vi "ListBox_MultiListBox.vi"() -> ()   [LabVIEW 2025]
doc: "Converts a 2D array into a multi-column listbox by using both the 'ItemNames' and 'Headers' property nodes, and also converts a 1D array into a listbox using the 'ItemNames' property node, allowing the user to select a value from the list, and displays the selected value."
panel:
  out "String":string
  out "Numeric":i32
  in  "Array 4":string[](array[string])
  in  "Listbox":i32[](listbox)
  in  "Multicolumn Listbox 2":i32(listbox)
  in  "Array 3":string[](array[string])
  in  "Array 2":string[][](array[string])
  in  "Array":string[][](array[string])
  out "Multicolumn Listbox":i32(listbox)
  # "Sample usage of multi column Listbox- Converting 2D array to Multicolumn listbox using Itemnames property node"
  # "Sample usage of multi column Listbox- Converting 2D array to Multicolumn listbox using ItemNames and headers property node"
  # "Sample usage of Listbox- Converting 1D array to  listbox using Itemnames property node and then allow user to select value and showing the selected value"
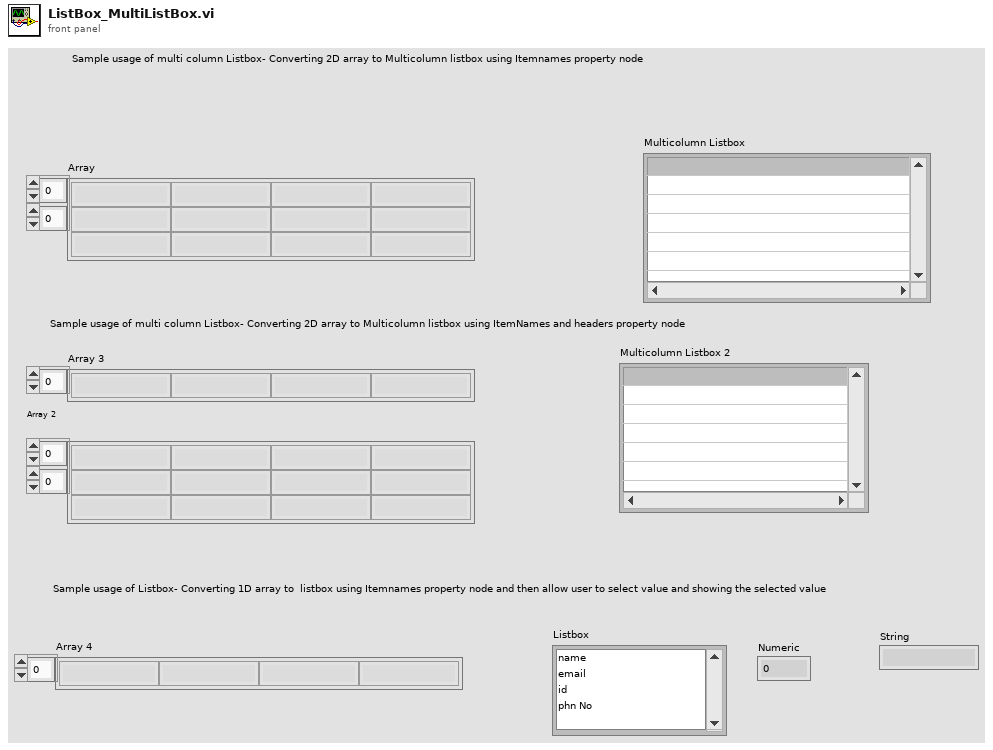
[diagram p1: front panel]
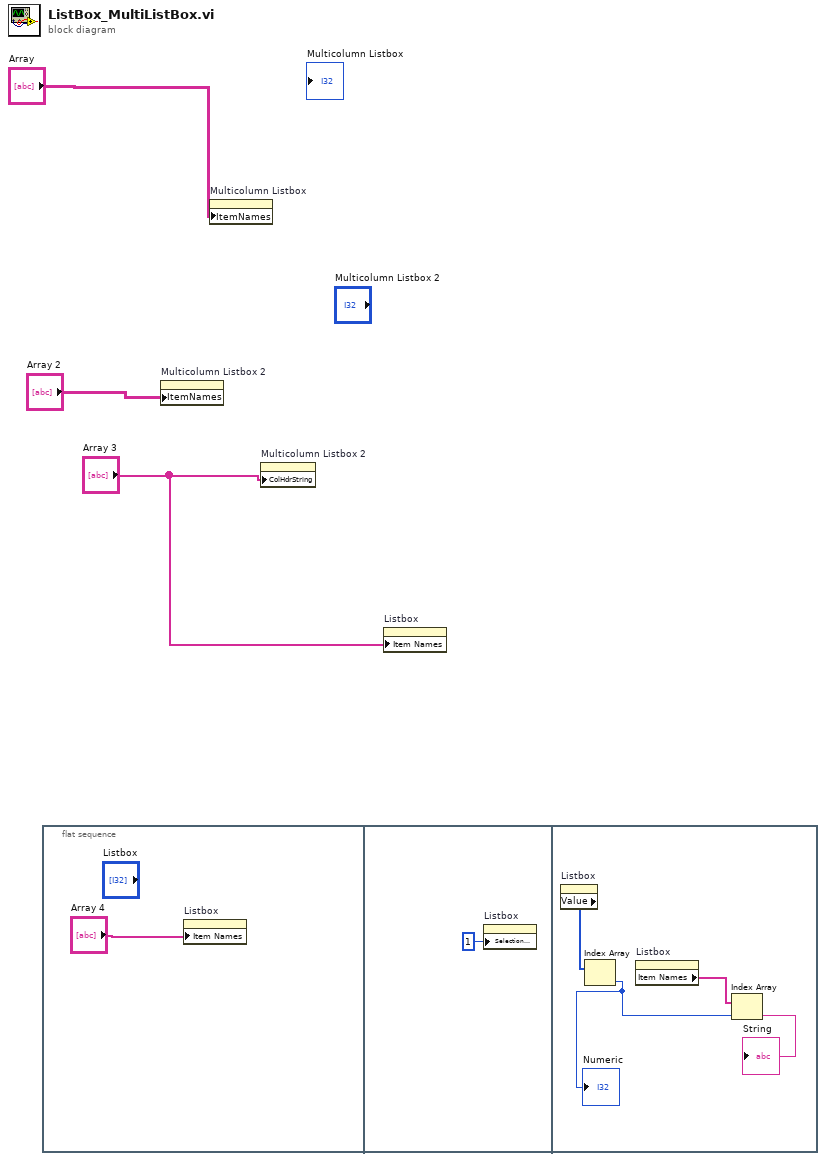
[diagram p0: block diagram]
diagram:
  n1 = flat-sequence {
    frame #0 {
      n2 = property on="Listbox" class="LstBox (strict)"("Item Names"="Array 4") -> ()  [unwired: 2 in, 2 out]
    }
    frame #1 {
      n3 = property on="Listbox" class="LstBox (strict)"("Selection Mode"=1) -> ()  [unwired: 2 in, 2 out]
    }
    frame #2 {
      n4 = property on="Listbox" class="LstBox (strict)"() -> ("Value"=w9:i32[])  [unwired: 2 in, 2 out]
      n5 = Index Array(array=w9) -> (element=w7:i32)  [unwired: 1 in]
      "Numeric" <- w7
      n6 = property on="Listbox" class="LstBox (strict)"() -> ("Item Names"=w8:string[])  [unwired: 2 in, 2 out]
      n7 = Index Array(array=w8, index=w7) -> (element=→"String":string)
    }
  }
  n8 = property on="Multicolumn Listbox 2" class="MCListbox (strict)"("ItemNames"="Array 2") -> ()  [unwired: 2 in, 2 out]
  n9 = property on="Multicolumn Listbox" class="MCListbox (strict)"("ItemNames"="Array") -> ()  [unwired: 2 in, 2 out]
  n10 = property on="Multicolumn Listbox 2" class="MCListbox (strict)"("ColHdrString"="Array 3") -> ()  [unwired: 2 in, 2 out]
  n11 = property on="Listbox" class="LstBox (strict)"("Item Names"="Array 3") -> ()  [unwired: 2 in, 2 out]
